vi "Prepare.vi"(8 "error in (no error)":errorcluster, 10 "Arguments":T1[](array[typedef]) {"Number" items=["? One or none"=0, "* Any"=-1, "+ At least one"=-2]}, 11 "LV Argument Parser in":refnum<class "LV Argument Parser.lvclass">) -> (0 "error out":errorcluster, 3 "LV Argument Parser out":refnum<class "LV Argument Parser.lvclass">)   [LabVIEW 2023, in "LV ArgParse.lvlib" / "LV Argument Parser.lvclass"]
uses:
  LV Argument Parser.lvclass
  Argument Definition.ctl
  LV Argument Parser.lvclass/LV Argument Parser.ctl
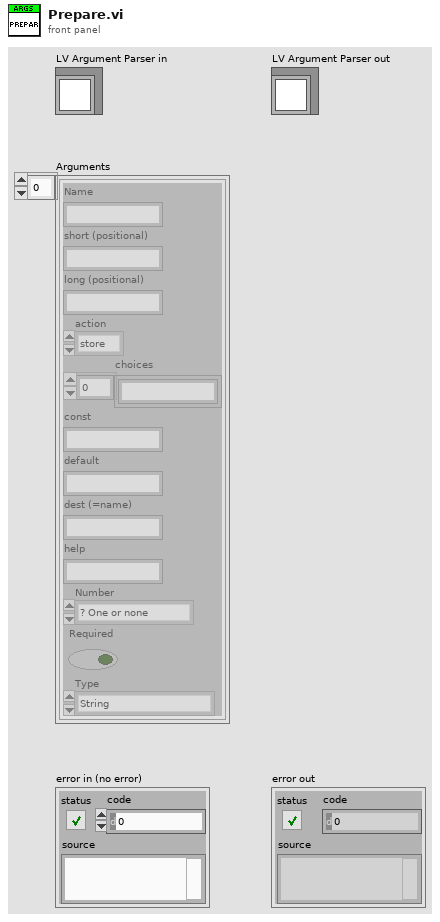
[diagram p1: front panel]
types:
  T1 = typedef "LV ArgParse.lvlib/LV Argument Parser.lvclass/Argument Definition.ctl" = cluster{"Name":string, "short (positional)":string, "long (positional)":string, "action":enum16{"store", "store-const", "store-false", "store-true", "append", "append-const", "count", "help", "version"}, "choices":string[], "const":string, "default":string, "dest (=name)":string, "help":string, "Number":i32, "Required":bool, "Type":enum16{"String", "Int", "Uint", "Float", "Bool", "Date", "Path"}}
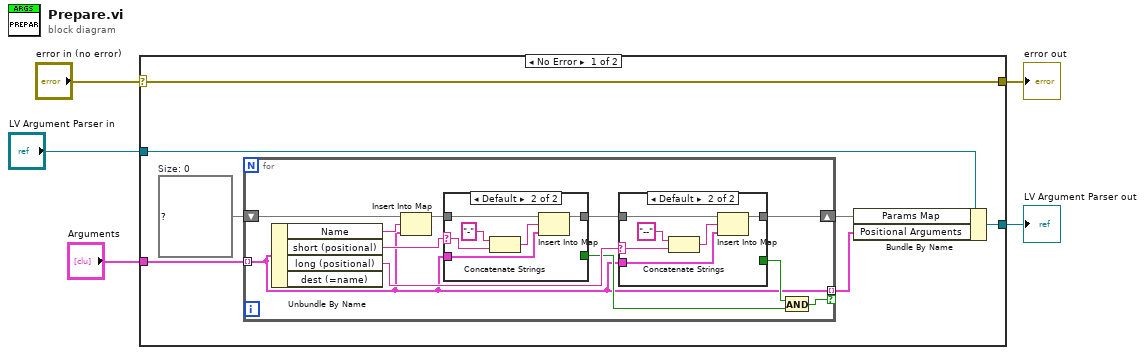
[diagram p0: block diagram]
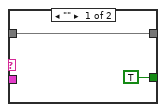
[diagram p2: hidden frame]
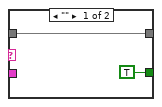
[diagram p3: hidden frame]
diagram:
  n1 = case shown="No Error" "error in (no error)" {
    selector: "error in (no error)" -> [w9 w40]
    tunnel: [w11 w41] -> w5
    tunnel: [w9 w40] -> w4
    tunnel: "LV Argument Parser in" -> [w7 w41]
    tunnel: "Arguments" -> [w6 _]
    frame No Error {
      w8 = map{string, T1} {}  # Size: 0
      n2 = for {
        tunnel: w6 -> [w13] mode=indexing
        tunnel: [w13] -> w12 mode=indexing if=w19
        shift-right: [w14] -> w10
        shift-left: w8 -> [w18]
        n3 = Unbundle By Name(w13) -> ("Name"=w17:string, "short (positional)"=w23:string, "long (positional)"=w22:string)  [unwired: 1 out]
        n4 = Insert Into Map(map in=w18, key=w17, value=w13) -> (map out=w16:map{string, T1})  [unwired: 2 out]
        n5 = case shown="Default" w23 {
          selector: w23 -> [_ w37]
          tunnel: w16 -> [w33 w39]
          tunnel: [w33 w38] -> w15
          tunnel: w13 -> [_ w36]
          tunnel: [TRUE _] -> w21
          frame "" {
          }
          frame Default {
            n6 = Concatenate Strings("-" ("string"), w37) -> (w35:string)
            n7 = Insert Into Map(map in=w39, key=w35, value=w36) -> (map out=w38:map{string, T1})  [unwired: 2 out]
          }
        }
        n8 = case shown="Default" w22 {
          selector: w22 -> [_ w29]
          tunnel: w15 -> [w25 w31]
          tunnel: [w25 w30] -> w14
          tunnel: w13 -> [_ w28]
          tunnel: [TRUE _] -> w20
          frame "" {
          }
          frame Default {
            n9 = Concatenate Strings("--" ("string"), w29) -> (w27:string)
            n10 = Insert Into Map(map in=w31, key=w27, value=w28) -> (map out=w30:map{string, T1})  [unwired: 2 out]
          }
        }
        n11 = And(x=w20, y=w21) -> (x .and. y?=w19:bool)
      }
      n12 = Bundle By Name(cluster=w7, "Params Map"=w10, "Positional Arguments"=w12) -> (w11:refnum<class "LV Argument Parser.lvclass">)
    }
    frame Error {
    }
  }
  "LV Argument Parser out" <- w5
  "error out" <- w4
